vi "Waveform Generation Loop.vi"(0 "Waveform Parameter FIFO":refnum<k33>, 5 "Debugging RT FIFO":refnum<k33>, 7 "DAQ Config Data":T1, 11 "error in (no error)":errorcluster) -> ()   [LabVIEW 2023, in "Waveform Analog Output Engine.lvlib"]
uses:
  Waveform Analog Output Engine.lvlib
  DAQ Config Data.ctl
  Console Message Type.ctl
  <vilib>/DAQmx/write.llb/DAQmx Write (Analog 1D Wfm NChan NSamp).vi
  Shared/Constants.vi
  <vilib>/DAQmx/miscellaneous.llb/DAQmx Fill In Error Info.vi
  <resource>/objmgr/daqmx.rc
  <vilib>/NI VeriStand/Custom Device Tools/Custom Device Utility Library/Custom Device Utility Library.lvlib
  Shared/Waveform Analog Output Shared.lvlib
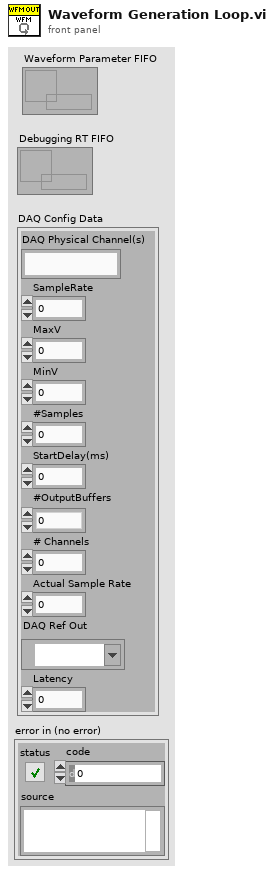
[diagram p1: front panel]
types:
  T1 = typedef "Waveform Analog Output Engine.lvlib/DAQ Config Data.ctl" = cluster{"DAQ Physical Channel(s)":string, "SampleRate":dbl, "MaxV":dbl, "MinV":dbl, "#Samples":dbl, "StartDelay(ms)":dbl, "#OutputBuffers":dbl, "# Channels":i32, "Actual Sample Rate":dbl, "DAQ Ref Out":refnum<k21>, "Latency":dbl}
  T2 = typedef "Waveform Analog Output Engine.lvlib/Console Message Type.ctl" = enum16{"Range Warning", "Error"}
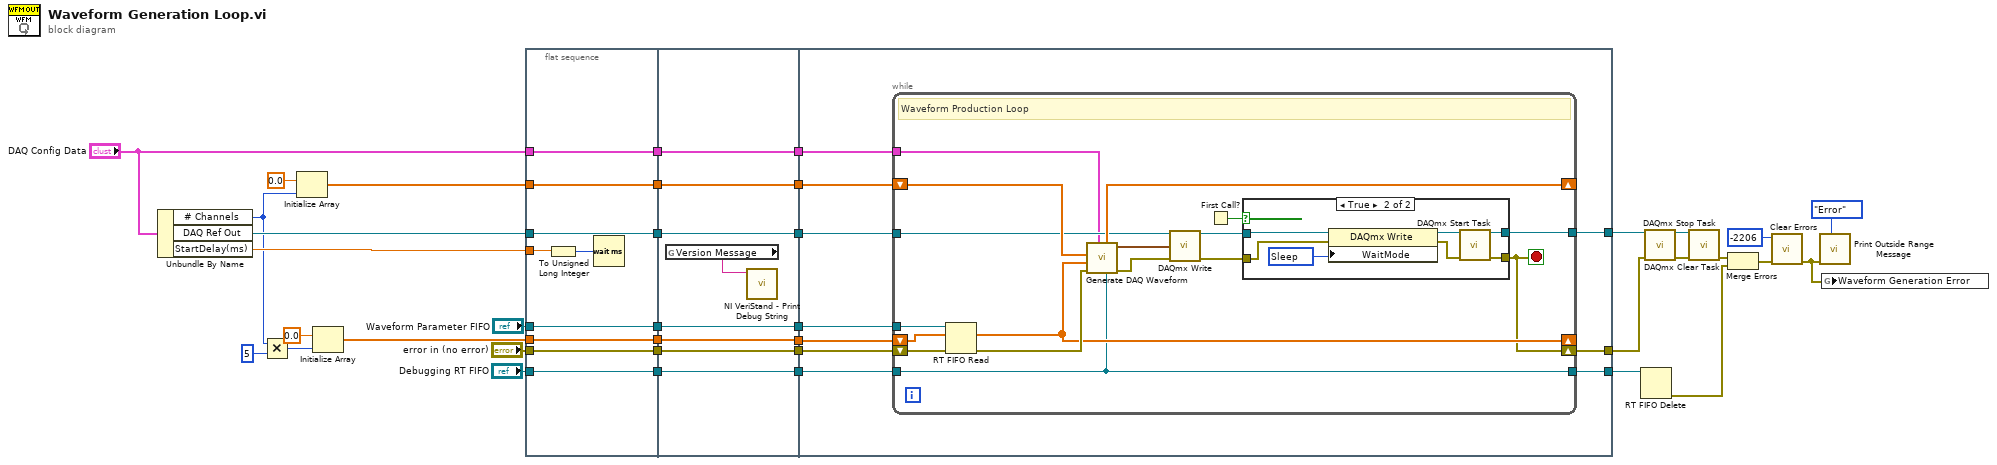
[diagram p0: block diagram]
diagram:
  n1 = Unbundle By Name("DAQ Config Data") -> ("# Channels"=w19:i32, "DAQ Ref Out"=w20:refnum<k21>, "StartDelay(ms)"=w23:dbl)
  n2 = Multiply(x=w19, y=5) -> (x*y=w16:i32)
  n3 = Initialize Array(0.0 ("element"), w19) -> (w21:dbl[])
  n4 = Initialize Array(0.0 ("element"), w16) -> (w15:dbl[])
  n5 = flat-sequence {
    tunnel: "Waveform Parameter FIFO" -> [w42]
    tunnel: w21 -> [w43]
    tunnel: w20 -> [w44]
    tunnel: "DAQ Config Data" -> [w45]
    tunnel: "error in (no error)" -> [w46]
    tunnel: "Debugging RT FIFO" -> [w47]
    tunnel: [w47] -> w30
    tunnel: [w46] -> w29
    tunnel: [w45] -> w28
    tunnel: [w44] -> w27
    tunnel: [w43] -> w26
    tunnel: [w42] -> w25
    tunnel: w23 -> [w40]
    tunnel: w15 -> [w39]
    tunnel: [w39] -> w14
    tunnel: [w55] -> w36
    tunnel: [w54] -> w35
    tunnel: [w53] -> w34
    tunnel: [w52] -> w33
    tunnel: [w51] -> w32
    tunnel: [w50] -> w31
    tunnel: w30 -> [w55]
    tunnel: w29 -> [w54]
    tunnel: w28 -> [w53]
    tunnel: w27 -> [w52]
    tunnel: w26 -> [w51]
    tunnel: w25 -> [w50]
    tunnel: w14 -> [w48]
    tunnel: [w48] -> w13
    tunnel: [w62] -> w8
    tunnel: [w61] -> w9
    tunnel: w36 -> [w65]
    tunnel: w35 -> [w64]
    tunnel: w34 -> [w63]
    tunnel: w33 -> [w60]
    tunnel: w32 -> [w59]
    tunnel: w31 -> [w58]
    tunnel: w13 -> [w57]
    tunnel: [w56] -> w7
    frame #0 {
      n6 = To Unsigned Long Integer(number=w40) -> (unsigned 32bit integer=w41:u32)
      n7 = Wait (ms)(milliseconds to wait=w41) -> ()  [unwired: 1 out]
    }
    frame #1 {
      n8 = global read "Constants.vi" "Version Message"() -> (w49:string)
      n9 = call <vilib>:"NI VeriStand - Print Debug String.vi"("Message"=w49) -> ()  [unwired: 10 in, 1 out]
    }
    frame #2 {
      n10 = while "Waveform Production Loop" {
        shift-right: [w67] -> w62
        shift-left: w64 -> [w71]
        tunnel: w58 -> [w72]
        shift-right: [w81] -> _
        shift-left: w59 -> [w82]
        tunnel: w60 -> [w74]
        tunnel: [w80] -> w61
        tunnel: w63 -> [w73]
        tunnel: w65 -> [w66]
        shift-right: [w68] -> _
        shift-left: w57 -> [w70]
        tunnel: [w66] -> w56
        stop <- w67 stop-if-true
        # "Waveform Production Loop"
        n11 = RT FIFO Read(0:w72, 1:w70, 3:w71) -> (9:w68:dbl[], 11:w69:errorcluster)  [unwired: 1 in, 3 out]
        n12 = call "Generate DAQ Waveform.vi"("Debug Message FIFO"=w66, "DAQ Config Data"=w73, "error in (no error)"=w69, "Channel Data"=w68, "Phase Array In"=w82) -> ("error out"=w76:errorcluster, "Waveform Array"=w75:waveform(dbl)[], "Phase Array Out out"=w81:dbl[])  [unwired: 4 in]
        n13 = call-poly <vilib>:"DAQmx Write.vi"("task/channels in"=w74, "data"=w75, "error in"=w76) -> ("task out"=w79:refnum<k21>, "error out"=w78:errorcluster)  [unwired: 10 in, 1 out]
        n14 = First Call?() -> (First Call?: T/F=w77:bool)
        n15 = case shown="True" w77 {
          tunnel: w79 -> [w83 w86]
          tunnel: w78 -> [w84 w85]
          tunnel: [w83 w90] -> w80
          tunnel: [w84 w89] -> w67
          frame False {
          }
          frame True {
            w91 = 12547 items=["Poll"=12524, "Yield"=12525, "Sleep"=12547] ("WaitMode")
            n16 = property class="DAQmx Write"(reference=w86, error in=w85, "WaitMode"=w91) -> (reference out=w88:refnum<k21>, error out=w87:errorcluster)
            n17 = call <vilib>:"DAQmx Start Task.vi"("task/channels in"=w88, "error in"=w87) -> ("task out"=w90:refnum<k21>, "error out"=w89:errorcluster)  [unwired: 12 in]
          }
        }
      }
    }
  }
  n18 = RT FIFO Delete(0:w7) -> (11:w5:errorcluster)  [unwired: 2 in]
  n19 = call <vilib>:"DAQmx Stop Task.vi"("task/channels in"=w9, "error in"=w8) -> ("task out"=w11:refnum<k21>, "error out"=w10:errorcluster)  [unwired: 12 in]
  n20 = call <vilib>:"DAQmx Clear Task.vi"("task in"=w11, "error in"=w10) -> ("error out"=w6:errorcluster)  [unwired: 13 in]
  n21 = Merge Errors(w6, w5) -> (w4:errorcluster)
  n22 = call <vilib>:"Clear Errors.vi"("error in (no error)"=w4, "specific error code to clear (0: all)"=-2206) -> ("error out"=w1:errorcluster)  [unwired: 4 in, 1 out]
  n23 = call "Print Outside Range Message.vi"("Message Type"=Console_Message_Type."Error", "error in (no error)"=w1) -> ()  [unwired: 10 in]
  n24 = global write "Constants.vi" "Waveform Generation Error"(w1) -> ()
